vi "_PC_Pub_XYPlot_Merge.vi"(8 "error in (no error)":errorcluster, 10 "Spectra":cluster{"X":dbl[], "Y":dbl[]}[](array[cluster])) -> (0 "error out":errorcluster, 2 "Spectrum out":cluster{"X":dbl[], "Y":dbl[]})   [LabVIEW 2018]
uses:
  <vilib>/gmath/NI_Gmath.lvlib
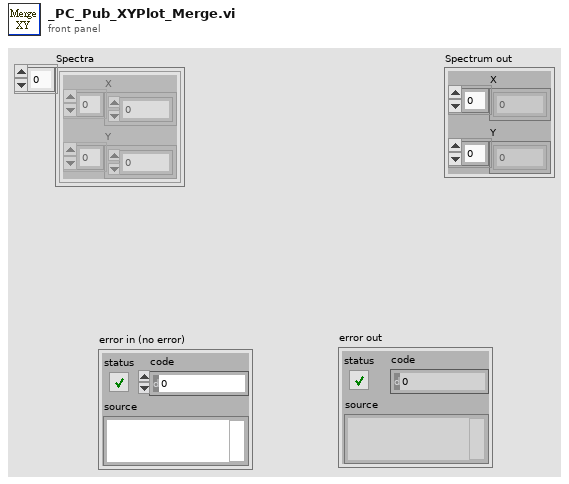
[diagram p1: front panel]
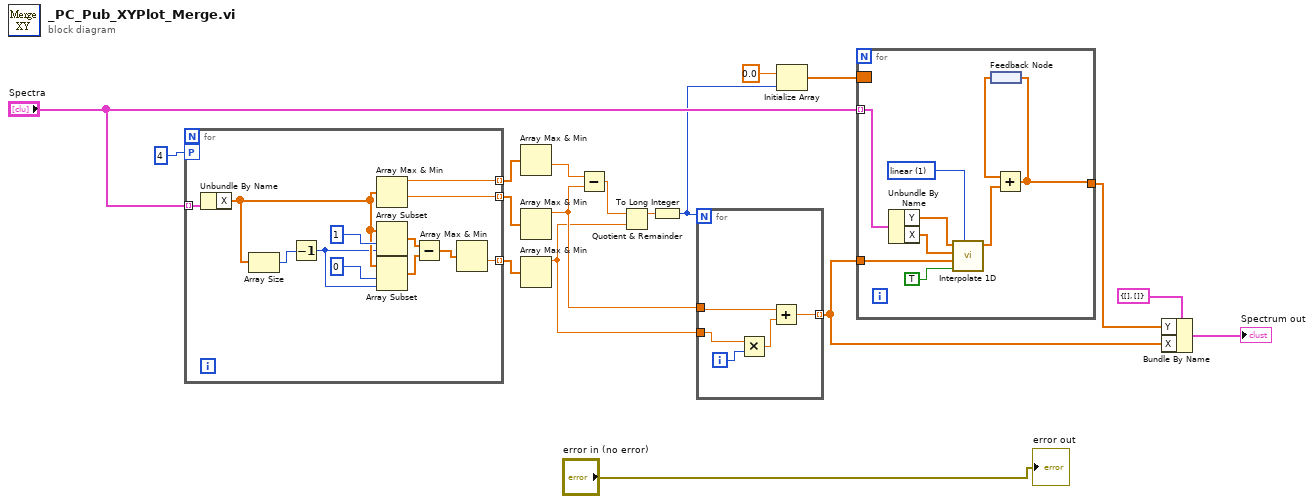
[diagram p0: block diagram]
diagram:
  n1 = for {
    tunnel: "Spectra" -> [w30] mode=indexing
    workers-P: 4 -> [_]
    tunnel: [w29] -> w17 mode=indexing
    tunnel: [w28] -> w16 mode=indexing
    tunnel: [w19] -> w15 mode=indexing
    n2 = Unbundle By Name(w30) -> ("X"=w25:dbl[])
    n3 = Array Size(array=w25) -> (size(s)=w26:i32)
    n4 = Decrement(x=w26) -> (x-1=w23:i32)
    n5 = Array Max & Min(array=w25) -> (max value=w29:dbl, min value=w28:dbl)  [unwired: 2 out]
    n6 = Array Subset(array=w25, index=1, length=w23) -> (w22:dbl[])
    n7 = Array Subset(array=w25, index=0, length=w23) -> (w21:dbl[])
    n8 = Subtract(x=w22, y=w21) -> (x-y=w20:dbl[])
    n9 = Array Max & Min(array=w20) -> (min value=w19:dbl)  [unwired: 3 out]
  }
  n10 = Array Max & Min(array=w17) -> (min value=w14:dbl)  [unwired: 3 out]
  n11 = Array Max & Min(array=w16) -> (max value=w11:dbl)  [unwired: 3 out]
  n12 = Array Max & Min(array=w15) -> (max value=w10:dbl)  [unwired: 3 out]
  n13 = Subtract(x=w14, y=w11) -> (x-y=w13:dbl)
  n14 = Quotient & Remainder(x=w13, y=w10) -> (floor(x/y)=w12:dbl)  [unwired: 1 out]
  n15 = To Long Integer(number=w12) -> (32bit integer=w8:i32)
  n16 = for {
    N: w8 -> [_]
    tunnel: w11 -> [w32]
    tunnel: w10 -> [w34]
    tunnel: [w31] -> w4 mode=indexing
    i -> [w35]
    n17 = Multiply(x=w34, y=w35) -> (x*y=w33:dbl)
    n18 = Add(x=w32, y=w33) -> (x+y=w31:dbl)
  }
  n19 = Initialize Array(0.0 ("element"), w8) -> (w6:dbl[])
  n20 = for {
    tunnel: "Spectra" -> [w42] mode=indexing
    tunnel: w4 -> [w44]
    border: w6 -> [_]
    tunnel: [w36] -> w3
    w39 = 1 items=["nearest", "linear", "spline", "cubic Hermite", "Lagrange"] ("method")
    n21 = Unbundle By Name(w42) -> ("Y"=w41:dbl[], "X"=w40:dbl[])
    n22 = call <vilib>:"Interpolate 1D.vi"("method"=w39, "X is monotonic"=TRUE, "xi"=w44, "X"=w40, "Y"=w41) -> ("yi"=w37:dbl[])  [unwired: 4 in, 2 out]
    n23 = feedback #1() -> (w38:dbl[])
    n24 = Add(x=w38, y=w37) -> (x+y=w36:dbl[])
    n25 = feedback-in #1(w36) -> ()
  }
  n26 = Bundle By Name(cluster=cluster{"X":dbl[], "Y":dbl[]} {"X"=[], "Y"=[]} ("Spectrum in"), "Y"=w3, "X"=w4) -> (→"Spectrum out":cluster{"X":dbl[], "Y":dbl[]})
  "error out" <- "error in (no error)"
